vi "LF Open File__ogtk.vi"(4 "error in (no error)":errorcluster, 5 "deny mode (2)":T1(ring)=enum."deny none", 6 "open mode (0)":T2(ring), 7 "file path":path) -> (0 "error out":errorcluster, 3 "refnum out":refnum<file>)   [LabVIEW 2014]
doc: "Opens a file for reading and or writing to. This function is very similar to the LabVIEW File Open fucntion but it does not resolve shortcuts to their target file location."
uses:
  kernel32.dll
panel:
  # "LF Open File.vi\n\nPlease visit http://www.OpenG.org to learn about the\nOpen Source LabVIEW software movement.\n\nNOTICE -- YOU MUST LEAVE THIS NOTICE IN PLACE.  PER THE TERMS OF THE LICENSE BELOW, YOU MAY SUBLICENSE THIS SOFTWARE \nIN ANY WAY THAT DOES NOT CONFLICT WITH THIS LICENSE.\n\n### BSD License (http://www.opensource.org/licenses/bsd-license.php) Begin ###\n\nCopyright (c) 2008, Rolf Kalbermatter <rolf.kalbermatter@citeng.com>\n\nAll rights reserved.\n\nRedistribution and use in source and binary forms, with or without modification, are permitted provided that the following conditions are met:\n\n    * Redistributions of source code must retain the above copyright notice, this list of conditions and the following disclaimer.\n    * Redistributions in binary form must reproduce the above copyright notice, this list of conditions and the following disclaimer in the \n       documentation and/or other materials provided with the distribution.\n    * Neither the name of SciWare, James Kring, Inc., nor the names of its contributors may be used to endorse or promote products derived \n       from this software without specific prior written permission.\n\nTHIS SOFTWARE IS PROVIDED BY THE COPYRIGHT HOLDERS AND CONTRIBUTORS \"AS IS\" AND ANY EXPRESS OR IMPLIED WARRANTIES, \nINCLUDING, BUT NOT LIMITED TO, THE IMPLIED WARRANTIES OF MERCHANTABILITY AND FITNESS FOR A PARTICULAR PURPOSE ARE \nDISCLAIMED. IN NO EVENT SHALL THE COPYRIGHT OWNER OR CONTRIBUTORS BE LIABLE FOR ANY DIRECT, INDIRECT, INCIDENTAL,\n SPECIAL, EXEMPLARY, OR CONSEQUENTIAL DAMAGES (INCLUDING, BUT NOT LIMITED TO, PROCUREMENT OF SUBSTITUTE GOODS OR \nSERVICES; LOSS OF USE, DATA, OR PROFITS; OR BUSINESS INTERRUPTION) HOWEVER CAUSED AND ON ANY THEORY OF LIABILITY, \nWHETHER IN CONTRACT, STRICT LIABILITY, OR TORT (INCLUDING NEGLIGENCE OR OTHERWISE) ARISING IN ANY WAY OUT OF THE USE \nOF THIS SOFTWARE, EVEN IF ADVISED OF THE POSSIBILITY OF SUCH DAMAGE.\n\n### BSD License End ###"
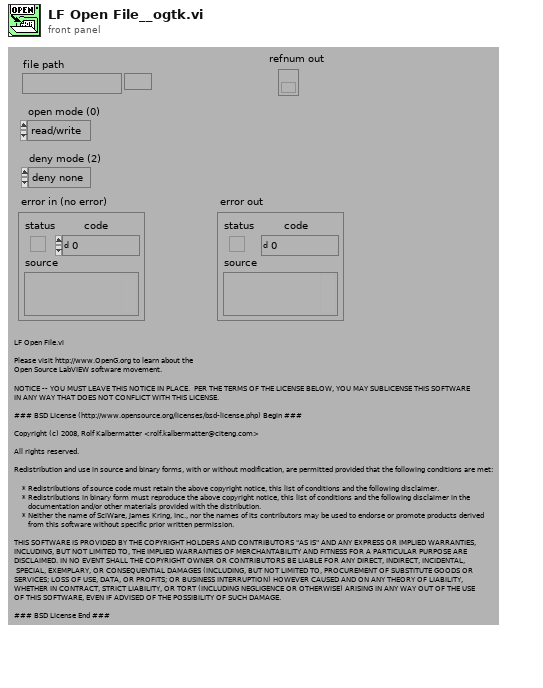
[diagram p1: front panel]
types:
  T1 = enum16{"deny read/write", "deny write-only", "deny none"}
  T2 = enum16{"read/write", "read-only", "write-only", "write-only (truncate)"}
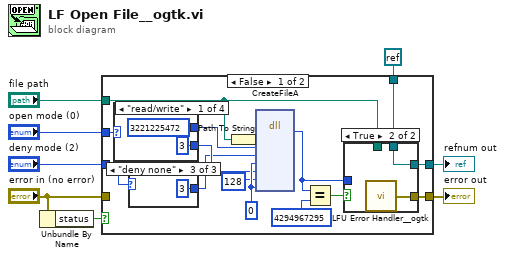
[diagram p0: block diagram]
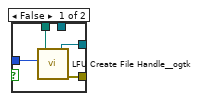
[diagram p2: hidden frame]
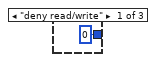
[diagram p3: hidden frame]
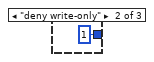
[diagram p4: hidden frame]
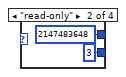
[diagram p5: hidden frame]
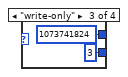
[diagram p6: hidden frame]
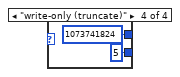
[diagram p7: hidden frame]
diagram:
  n1 = Unbundle By Name("error in (no error)") -> ("status"=w8:bool)
  n2 = case shown="False" w8 {
    tunnel: "error in (no error)" -> [_ w42]
    tunnel: [w15 w42] -> w6
    tunnel: "file path" -> [w13 _]
    tunnel: "open mode (0)" -> [w21 _]
    tunnel: "deny mode (2)" -> [w18 _]
    tunnel: [w14 w41] -> w2
    tunnel: refnum<k0> refnum -> [w9 w41]
    frame False {
      w22 = u32 0 ("TemplateFile")
      n3 = case shown="\"read/write\"" w21 {
        tunnel: [u32 3221225472 u32 2147483648 u32 1073741824 u32 1073741824] -> w20
        tunnel: [u32 3 u32 3 u32 3 u32 5] -> w19
        frame "read/write" {
        }
        frame "read-only" {
        }
        frame "write-only" {
        }
        frame "write-only (truncate)" {
        }
      }
      n4 = case shown="\"deny none\"" w18 {
        tunnel: [u32 0 u32 1 u32 3] -> w17
        frame "deny read/write" {
        }
        frame "deny write-only" {
        }
        frame "deny none" {
        }
      }
      n5 = Path To String(path=w13) -> (string=w23:string)
      n6 = dll-call lib="kernel32.dll" fn="CreateFileA"("fileName"=w23, "desiredAccess"=w20, "shareMode"=w17, "securityDesc"=w22, "creationDisposition"=w19, "flagsAttributes"=u32 128, "TemplateFile"=w22) -> (w11:u32)  [unwired: 10 in, 2 out]
      n7 = Equal?(x=w11, y=u32 4294967295 ("retval")) -> (x = y?=w10:bool)
      n8 = case shown="True" w10 {
        tunnel: [w25 w28] -> w15
        tunnel: [w24 w29] -> w14
        tunnel: w13 -> [w26 _]
        tunnel: w11 -> [w27 _]
        tunnel: w9 -> [_ w29]
        frame False {
          n9 = call <userlib>:"LFU Create File Handle__ogtk.vi"("handle"=w27, "file path"=w26) -> ("error out"=w25:errorcluster, "file refnum"=w24:refnum<file>)  [unwired: 4 in]
        }
        frame True {
          n10 = call <userlib>:"LFU Error Handler__ogtk.vi"() -> ("error out"=w28:errorcluster)  [unwired: 2 in]
        }
      }
    }
    frame True {
    }
  }
  "refnum out" <- w2
  "error out" <- w6
